vi "Read XML_Extra Checks_Check BCD Parameters Bits Settings.vi"(8 "error in (no error)":errorcluster, 11 "Channels In":T1[](array[typedef])) -> (0 "error out":errorcluster)   [LabVIEW 2019]
doc: "This VI checks that for a given Hardware Channel, all parameters have a unique combination of Parameter settings: Hardware Channel, Label Decimal and Parameter Name. If there are multiple duplicates, the function returns all duplicates."
uses:
  XML_Channel.ctl
  XML_Label.ctl
  XML_Parameter.ctl
  <userlib>/_OpenG.lib/array/array.llb/Filter 1D Array with Scalar (Boolean)__ogtk.vi
panel:
  out "Error Source":string
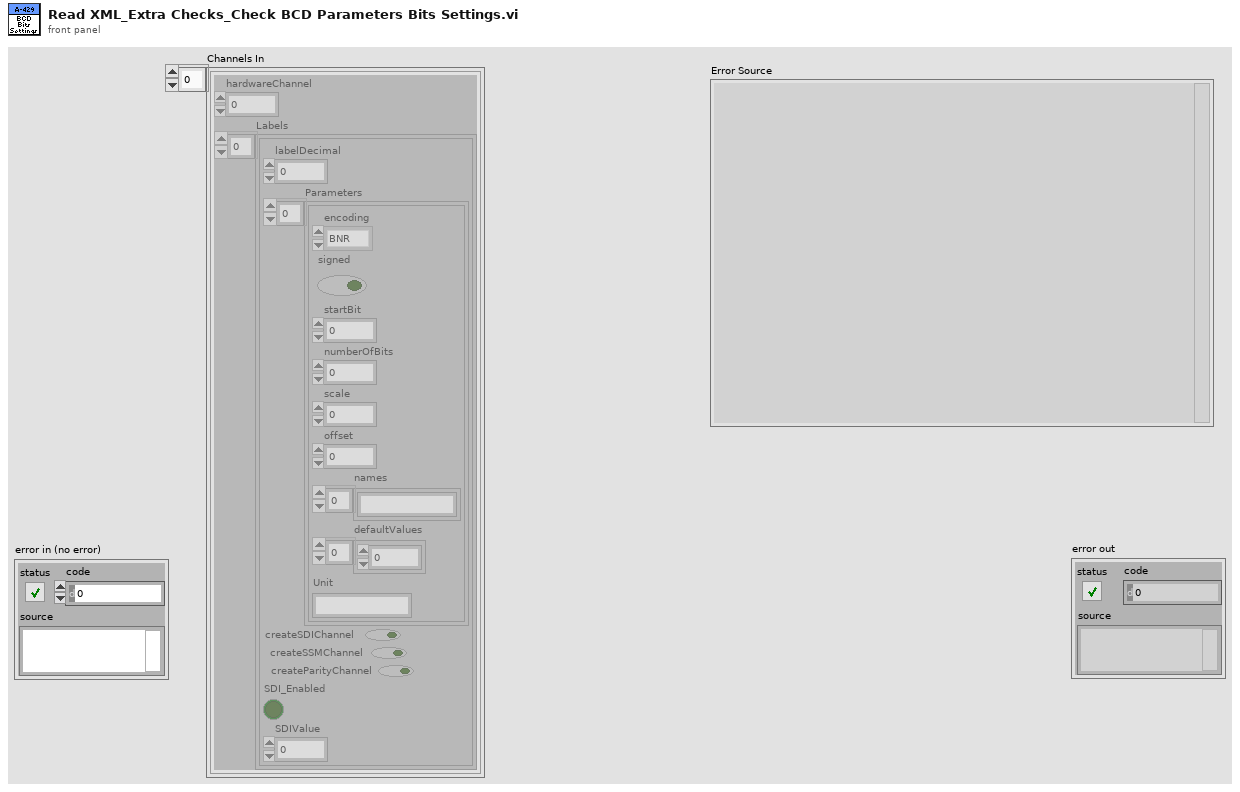
[diagram p1: front panel]
types:
  T1 = typedef "XML_Channel.ctl" = cluster{"hardwareChannel":i32, "Labels":T2[]}
  T2 = typedef "XML_Label.ctl" = cluster{"labelDecimal":i32, "Parameters":T3[], "createSDIChannel":bool, "createSSMChannel":bool, "createParityChannel":bool, "SDI_Enabled":bool, "SDIValue":u8}
  T3 = typedef "XML_Parameter.ctl" = cluster{"encoding":enum16{"BNR", "BCD", "Discrete"}, "signed":bool, "startBit":i32, "numberOfBits":i32, "scale":dbl, "offset":dbl, "names":string[], "defaultValues":dbl[], "Unit":string}
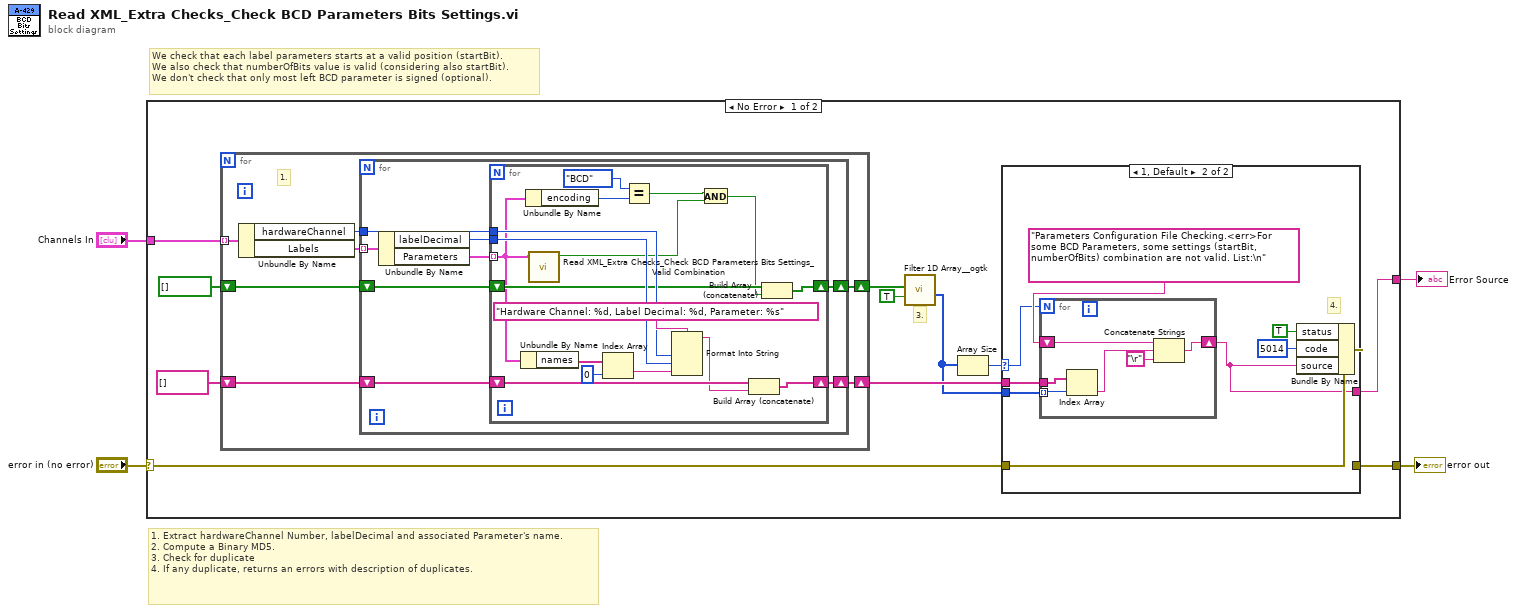
[diagram p0: block diagram]
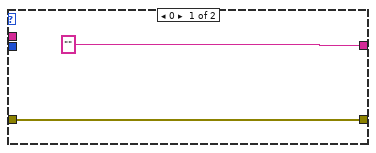
[diagram p2: hidden frame]
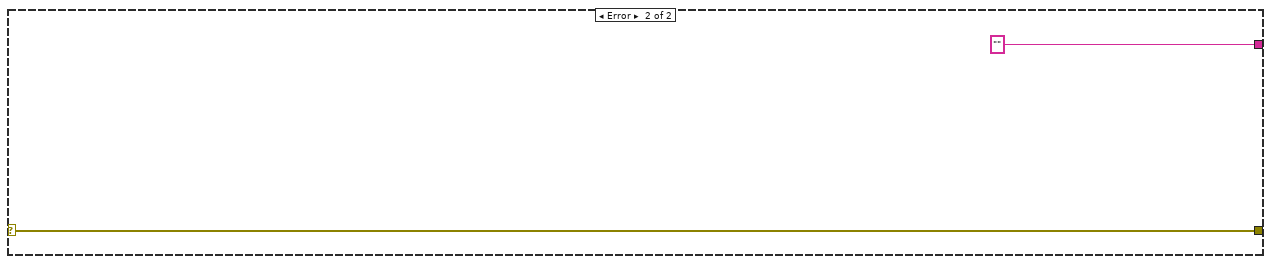
[diagram p3: hidden frame]
diagram:
  # "We check that each label parameters starts at a valid position (startBit).\nWe also check that numberOfBits value is valid (considering also startBit).\nWe don't check that only most left BCD parameter is signed (optional)."
  # "1. Extract hardwareChannel Number, labelDecimal and associated Parameter's name.\n2. Compute a Binary MD5.\n3. Check for duplicate\n4. If any duplicate, returns an errors with description of duplicates."
  n1 = case shown="No Error" "error in (no error)" {
    selector: "error in (no error)" -> [w14 w66]
    tunnel: [w12 w66] -> w3
    tunnel: "Channels In" -> [w13 _]
    tunnel: [w11 ""] -> w1
    frame No Error {
      # "3."
      n2 = for {
        tunnel: w13 -> [w39] mode=indexing
        shift-right: [w35] -> w8
        shift-left: bool[] [] -> [w36]
        shift-right: [w33] -> w9
        shift-left: string[] [] -> [w34]
        # "1."
        n3 = Unbundle By Name(w39) -> ("hardwareChannel"=w38:i32, "Labels"=w37:T2[])
        n4 = for {
          tunnel: w38 -> [w47]
          tunnel: w37 -> [w46] mode=indexing
          shift-right: [w43] -> w35
          shift-left: w36 -> [w44]
          shift-right: [w40] -> w33
          shift-left: w34 -> [w41]
          n5 = Unbundle By Name(w46) -> ("labelDecimal"=w45:i32, "Parameters"=w42:T3[])
          n6 = for {
            tunnel: w47 -> [w59]
            tunnel: w45 -> [w64]
            shift-right: [w58] -> w43
            shift-left: w44 -> [w57]
            tunnel: w42 -> [w49] mode=indexing
            shift-right: [w62] -> w40
            shift-left: w41 -> [w63]
            n7 = Unbundle By Name(w49) -> ("names"=w52:string[])
            n8 = Unbundle By Name(w49) -> ("encoding"=w56:enum16{"BNR", "BCD", "Discrete"})
            n9 = call "Read XML_Extra Checks_Check BCD Parameters Bits Settings_Valid Combination.vi"("Parameter"=w49) -> ("Not Valid"=w48:bool)  [unwired: 10 in]
            n10 = Index Array(array=w52, index=0) -> (element=w50:string)
            n11 = Equal?(x=enum16{"BNR", "BCD", "Discrete"}."BCD", y=w56) -> (x = y?=w54:bool)
            n12 = Format Into String(format string="Hardware Channel: %d, Label Decimal: %d, Parameter: %s", w59, w64, w50) -> (resulting string=w60:string)  [unwired: 2 in, 1 out]
            n13 = And(x=w54, y=w48) -> (x .and. y?=w53:bool)
            n14 = Build Array (concatenate)(w63, w60) -> (w62:string[])
            n15 = Build Array (concatenate)(w57, w53) -> (w58:bool[])
          }
        }
      }
      n16 = call-poly <userlib>:"Filter 1D Array__ogtk.vi"("items to filter"=TRUE, "array"=w8) -> ("filtered item indices"=w7:i32[])  [unwired: 4 in, 1 out]
      n17 = Array Size(array=w7) -> (size(s)=w15:i32)
      n18 = case shown="1, Default" w15 {
        selector: w15 -> [_ w21]
        tunnel: w14 -> [w17 w26]
        tunnel: w7 -> [_ w20]
        tunnel: [w17 w25] -> w12
        tunnel: ["" w19] -> w11
        tunnel: w9 -> [_ w18]
        frame 0 {
        }
        frame 1, Default {
          # "4."
          n19 = for {
            N: w21 -> [_]
            shift-right: [w31] -> w19
            shift-left: "Parameters Configuration File Checking.<err>For some BCD Parameters, some settings (startBit, numberOfBits) combination are not valid. List:\n" -> [w32]
            tunnel: w20 -> [w30] mode=indexing
            tunnel: w18 -> [w28]
            n20 = Index Array(array=w28, index=w30) -> (element=w27:string)
            n21 = Concatenate Strings(w32, w27, "\r") -> (w31:string)
          }
          n22 = Bundle By Name(cluster=w26, "status"=TRUE, "code"=5014, "source"=w19) -> (w25:errorcluster)
        }
      }
    }
    frame Error {
    }
  }
  "error out" <- w3
  "Error Source" <- w1
